vi "Build experiment folder path.vi"(8 "error in (no error)":errorcluster, 11 "Experiment folder base name":T1) -> (0 "error out":errorcluster, 3 "Experiment folder  file path":path)   [LabVIEW 2017]
uses:
  Logging/Typedefs/Experiment folder base name.ctl
  Global Variables/gl_UI Ctrl Refs.vi
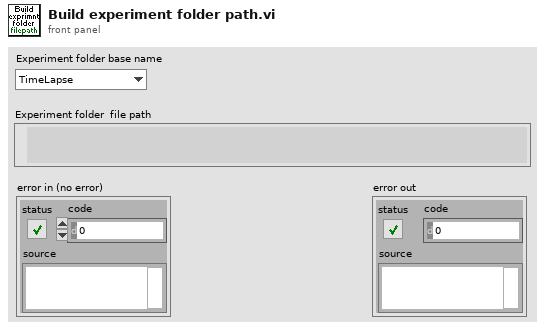
[diagram p1: front panel]
types:
  T1 = typedef "Experiment folder base name.ctl" = enum16{"TimeLapse", "FunctAcq"}
  T2 = typedef "UI ctrl refs cluster.ctl" = cluster{"Top level VI path":path, "Top level VI ref":refnum<vi>, "User menu ref":refnum<k9>, "Sub Panel control":refnum<vi>, "Imaging Param Tab":refnum<vi>, "Occurrence-Start drivers":refnum<k4>, "Occurrence-Speed logging initialised":refnum<k4>, "Occurrence-XYZ stage initialised":refnum<k4>, "Exit button":refnum<vi>, "Status ind":refnum<vi>, "Set as origin":refnum<vi>, "Speed Logging":refnum<vi>, "Time Lapse":refnum<vi>, "Live Imaging":refnum<vi>, "AOL Z Stack":refnum<vi>, "Motor Z Stack":refnum<vi>, "Funct Acq button":refnum<vi>, "Hard Shutter":refnum<vi>, "Virtual Shutter":refnum<vi>, "Laser Power":refnum<vi>, "AOL Mode":refnum<vi>, "Frame Size":refnum<vi>, "Field of View":refnum<vi>, "Dwell Time":refnum<vi>, "Zoom":refnum<vi>, "AOL Z":refnum<vi>, "Objective":refnum<vi>, "Axis":refnum<vi>, "Paths & Names":refnum<vi>, "Experiment folder path (ind.)":refnum<vi>, "Last State (Ind.)":refnum<vi>, "Laser wavelength ind (nm)":refnum<vi>, "Averages":refnum<vi>, "Angle (degrees)":refnum<vi>, "X centre":refnum<vi>, "Y centre":refnum<vi>, "Plane Mode":refnum<vi>, "# Planes":refnum<vi>, "Z Start":refnum<vi>, "Z Stop":refnum<vi>, "Z Step":refnum<vi>, "PMT 1":refnum<vi>, "PMT 2":refnum<vi>, "Stage XYZ Position":refnum<vi>, "Pockels@Z Start":refnum<vi>, "Pockels@Z Stop":refnum<vi>, "Obtain Z Start":refnum<vi>, "Obtain Z Stop":refnum<vi>, "Live stim.trig.period":refnum<vi>, "Live stim.trig.enable":refnum<vi>, "Movement Correction":refnum<vi>, "Load Reference Image":refnum<vi>, "XY Stage Move":refnum<vi>, "MovCor Cluster":refnum<vi>, "RefDAQParam":refnum<vi>, "Funct. Acq. Pockels Modulation":refnum<vi>, "Background MovCor":refnum<vi>, "Ref Laser Power":refnum<vi>, "Enable Video Recording":refnum<vi>, "Video Record-Live Imaging":refnum<vi>, "Video Record-Funct acq":refnum<vi>, "Reference Source":refnum<vi>, "AOL Z-stack Chirps Ready (ind)":refnum<vi>, "Target time between mov.cor. ref triggers (ms)":refnum<vi>, "Funct. Acq. Ref frame save":refnum<vi>, "Tracking button":refnum<vi>, "Show ref plots window":refnum<vi>, "Center freq ind (nm)":refnum<vi>, "Pickup mode (ind)":refnum<vi>, "Logging queue (ind)":refnum<vi>, "Back aperture power (ind.)":refnum<vi>, "Power after objective (ind.)":refnum<vi>, "Switch user":refnum<vi>}
  T3 = cluster{"Base Directory":path, "User folder?":bool, "Sub-Folder":string, "Experiment folder custom name":string}
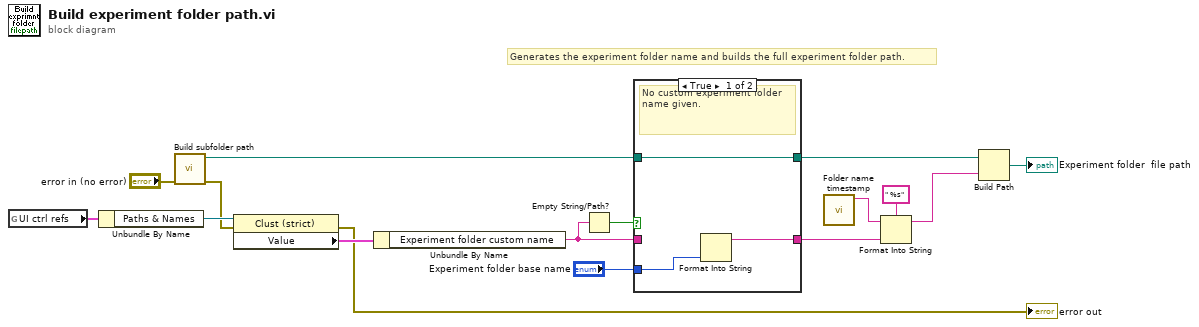
[diagram p0: block diagram]
diagram:
  # "Generates the experiment folder name and builds the full experiment folder path."
  n1 = global read "gl_UI Ctrl Refs.vi" "UI ctrl refs"() -> (w15:T2)
  n2 = Unbundle By Name(w15) -> ("Paths & Names"=w14:refnum<vi>)
  n3 = call "Build subfolder path.vi"("error in (no error)"="error in (no error)") -> ("error out"=w9:errorcluster, "Daily folder or sub-folder path"=w11:path)  [unwired: 9 in]
  n4 = property on="Property Node" class="Clust (strict)"(reference=w14, error in=w9) -> (error out=→"error out":errorcluster, "Value"=w16:T3)  [unwired: 1 out]
  n5 = Unbundle By Name(w16) -> ("Experiment folder custom name"=w13:string)
  n6 = Empty String/Path?(string/path=w13) -> (empty?=w12:bool)
  n7 = case shown="True" w12 {
    tunnel: w11 -> [w17 w21]
    tunnel: w13 -> [_ w20]
    tunnel: [w17 w21] -> w3
    tunnel: "Experiment folder base name" -> [w19 _]
    tunnel: [w18 w20] -> w1
    frame True {
      # "No custom experiment folder name given."
      n8 = Format Into String(w19) -> (resulting string=w18:string)  [unwired: 3 in, 1 out]
    }
    frame False {
      # "Custom experiment folder name given."
    }
  }
  n9 = call "Folder name timestamp.vi"() -> ("date/time string"=w6:string)  [unwired: 11 in]
  n10 = Format Into String(format string=" %s" ("name or relative path"), initial string=w6, w1) -> (resulting string=w4:string)  [unwired: 1 in, 1 out]
  n11 = Build Path(base path=w3, name or relative path=w4) -> (appended path=→"Experiment folder  file path":path)
